vi "Setup Measurement.vi"(8 "error in (no error)":errorcluster, 10 "Window Handle":i32, 11 "Config File Path":path=path "TestStand.ini") -> (0 "error out":errorcluster, 1 "Show UI?":bool, 2 "Device Names":string[](array[string]), 3 "Measurement Name":string)   [LabVIEW 2015, in "TestStand API.lvlib"]
uses:
  TestStand API.lvlib
  Measurement Setup/Measurement Setup.lvclass
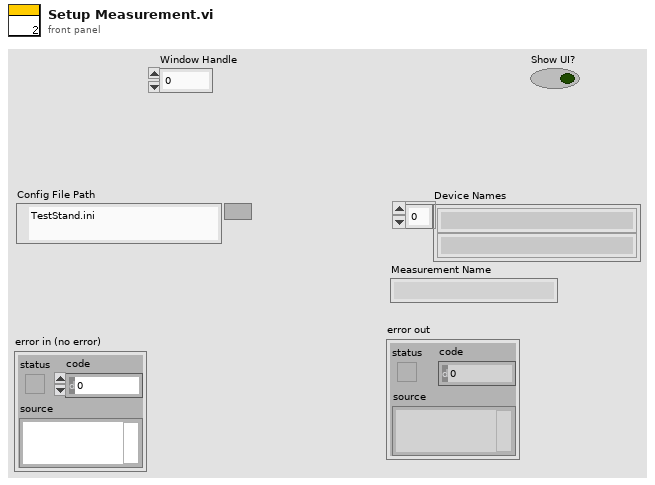
[diagram p1: front panel]
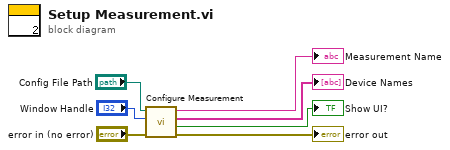
[diagram p0: block diagram]
diagram:
  n1 = call "Configure Measurement.vi"("error in (no error)"="error in (no error)", "Window Handle"="Window Handle", "Config File Path"="Config File Path") -> ("error out"=→"error out":errorcluster, "Show UI?"=→"Show UI?":bool, "Device Names"=→"Device Names":string[], "Measurement Name"=→"Measurement Name":string)  [unwired: 5 in]
